vi "zad5.vi"() -> ()   [LabVIEW 2018]
uses:
  <vilib>/DAQmx/read.llb/DAQmx Read (Analog 1D Wfm NChan NSamp).vi
  <vilib>/DAQmx/create/channels.llb/DAQmx Create Channel (AI-Acceleration-Accelerometer).vi
  <vilib>/DAQmx/configure/timing.llb/DAQmx Timing (Sample Clock).vi
  <vilib>/DAQmx/miscellaneous.llb/DAQmx Fill In Error Info.vi
panel:
  in  "file path":path
  in  "?":bool
  out "Time Signal":waveform(dbl)[](graph)
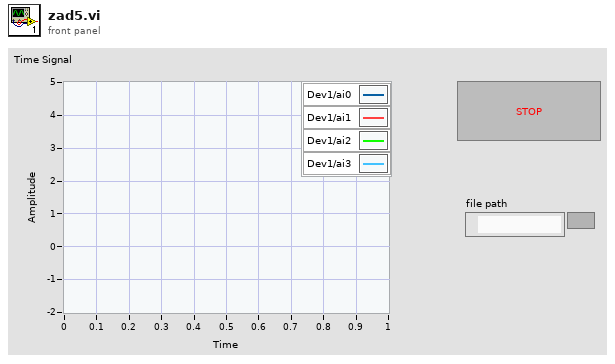
[diagram p1: front panel]
types:
  T1 = enum16{"open", "open or create", "create or replace", "create", "open (read-only)"}
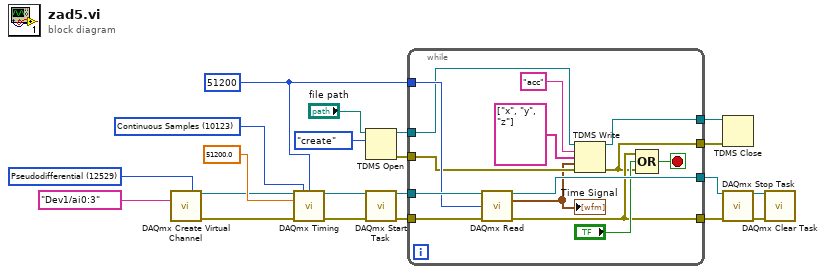
[diagram p0: block diagram]
diagram:
  w7 = 12529 items=["default"=-1, "RSE"=10083, "NRSE"=10078, "Differential"=10106, "Pseudodifferential"=12529] ("input terminal configuration")
  w12 = 51200 ("samples per channel")
  w18 = 10123 items=["Finite Samples"=10178, "Continuous Samples"=10123, "Hardware Timed Single Point"=12522] ("sample mode")
  n1 = call-poly <vilib>:"DAQmx Create Virtual Channel.vi"("input terminal configuration"=w7, "physical channels"=tag "Dev1/ai0:3") -> ("task out"=w17:refnum<k21>, "error out"=w20:errorcluster)  [unwired: 12 in]
  n2 = call-poly <vilib>:"DAQmx Timing.vi"("task/channels in"=w17, "sample mode"=w18, "samples per channel"=w12, "rate"=51200.0, "error in"=w20) -> ("task out"=w16:refnum<k21>, "error out"=w15:errorcluster)  [unwired: 9 in]
  n3 = TDMS Open(10:T1."create" ("operation (0:open)"), 11:"file path") -> (0:w4:errorcluster, 3:w6:refnum<k34>)  [unwired: 5 in]
  n4 = call <vilib>:"DAQmx Start Task.vi"("task/channels in"=w16, "error in"=w15) -> ("task out"=w14:refnum<k21>, "error out"=w13:errorcluster)  [unwired: 12 in]
  n5 = while {
    tunnel: w14 -> [w35]
    tunnel: w13 -> [w34]
    tunnel: w12 -> [w29]
    tunnel: [w33] -> w11
    tunnel: [w31] -> w10
    tunnel: w6 -> [w28]
    tunnel: [w27] -> w5
    tunnel: w4 -> [w26]
    tunnel: [w25] -> w3
    stop <- w30 stop-if-true
    n6 = call-poly <vilib>:"DAQmx Read.vi"("task/channels in"=w35, "number of samples per channel"=w29, "error in"=w34) -> ("task out"=w33:refnum<k21>, "data"=w24:waveform(dbl)[], "error out"=w31:errorcluster)  [unwired: 10 in]
    "Time Signal" <- w24
    n7 = TDMS Write(0:w28, 5:"acc" ("group name in (Untitled)"), 7:string[] ["x", "y", "z"] ("channel name(s) in (Untitled)"), 9:w24, 11:w26) -> (4:w27:refnum<k34>, 15:w25:errorcluster)  [unwired: 1 in, 2 out]
    n8 = Compound Arithmetic op=OR(w31, "?", w25) -> (w30:bool)
  }
  n9 = TDMS Close(8:w3, 11:w5) -> ()  [unwired: 2 out]
  n10 = call <vilib>:"DAQmx Stop Task.vi"("task/channels in"=w11, "error in"=w10) -> ("task out"=w9:refnum<k21>, "error out"=w8:errorcluster)  [unwired: 12 in]
  n11 = call <vilib>:"DAQmx Clear Task.vi"("task in"=w9, "error in"=w8) -> ()  [unwired: 13 in, 1 out]
